vi "Write Analogue.vi"(8 "error in (no error)":errorcluster, 9 "Outbput":bool, 10 "Channel index(0)":i32, 11 "APS 7050":refnum<class "APS 7050.lvclass">) -> (0 "error out":errorcluster, 2 "Success?":bool, 3 "APS 7050 out":refnum<class "APS 7050.lvclass">)   [LabVIEW 2025, in "Power Supply.lvlib" / "APS 7050.lvclass"]
uses:
  APS 7050.lvclass
  APS 7050.lvclass/APS 7050.ctl
  <instrlib>/APS-7000 Series/APS-7000 Series.lvlib
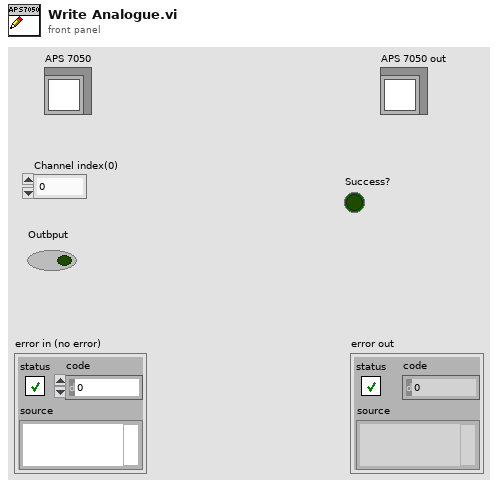
[diagram p1: front panel]
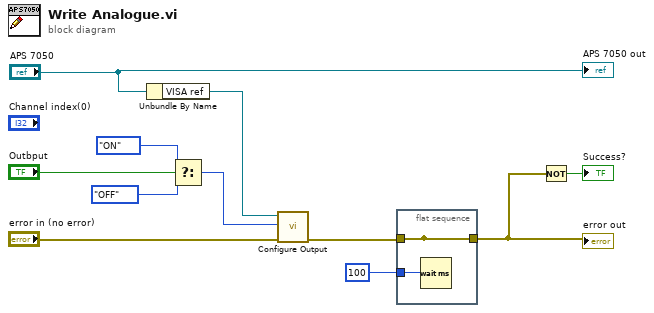
[diagram p0: block diagram]
diagram:
  n1 = Unbundle By Name("APS 7050") -> ("VISA ref"=w6:refnum<visa-resource-name>)
  n2 = Select(t=enum16{"OFF", "ON"}."ON" ("Output ON/OFF"), s="Outbput", f=enum16{"OFF", "ON"}."OFF" ("Output ON/OFF")) -> (s? t:f=w7:enum16{"OFF", "ON"})
  n3 = call <instrlib>:"Configure Output.vi"("error in"="error in (no error)", "Output ON/OFF"=w7, "VISA in"=w6) -> ("error out"=w5:errorcluster)  [unwired: 6 in, 2 out]
  n4 = flat-sequence {
    tunnel: [w12] -> _
    tunnel: w5 -> [w12]
    tunnel: u32 100 ("milliseconds to wait") -> [w13]
    tunnel: [w12] -> w3
    frame #0 {
      n5 = Wait (ms)(milliseconds to wait=w13) -> ()  [unwired: 1 out]
    }
  }
  n6 = Not(x=w3) -> (.not. x?=→"Success?":bool)
  "error out" <- w3
  "APS 7050 out" <- "APS 7050"
